vi "Set ComboCell DataSource.vi"   [LabVIEW 2016, in "DataGrid.lvlib" / "DataGridView.lvclass"]
uses:
  <userlib>/LabVIEWdotNetDataGrid/source/DataGridView/DataGridView.lvclass
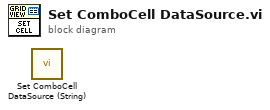
[diagram p0: block diagram]
diagram:
  n1 = call <userlib>:"Set ComboCell DataSource (String).vi"() -> ()  [unwired: 14 in, 2 out]
